vi "MoveROI.vi"(7 "Direction":enum16{"X+", "X-", "Y+", "Y-"}(ring), 8 "error in (no error)":errorcluster, 9 "Pitch":i32, 10 "ROI In":T1 {"Contours"."Type" items=["No Selection", "Point", "Line", "Rectangle", "Oval", "Polygon", "Freehand Region", "Annulus", "Unused2", "Unused3", "Broken Line", "Freehand Line", "Rotated Rectangle"]}) -> (0 "error out":errorcluster, 2 "ROI Out":T1 {"Contours"."Type" items=["No Selection", "Point", "Line", "Rectangle", "Oval", "Polygon", "Freehand Region", "Annulus", "Unused2", "Unused3", "Broken Line", "Freehand Line", "Rotated Rectangle"]})   [LabVIEW 2019]
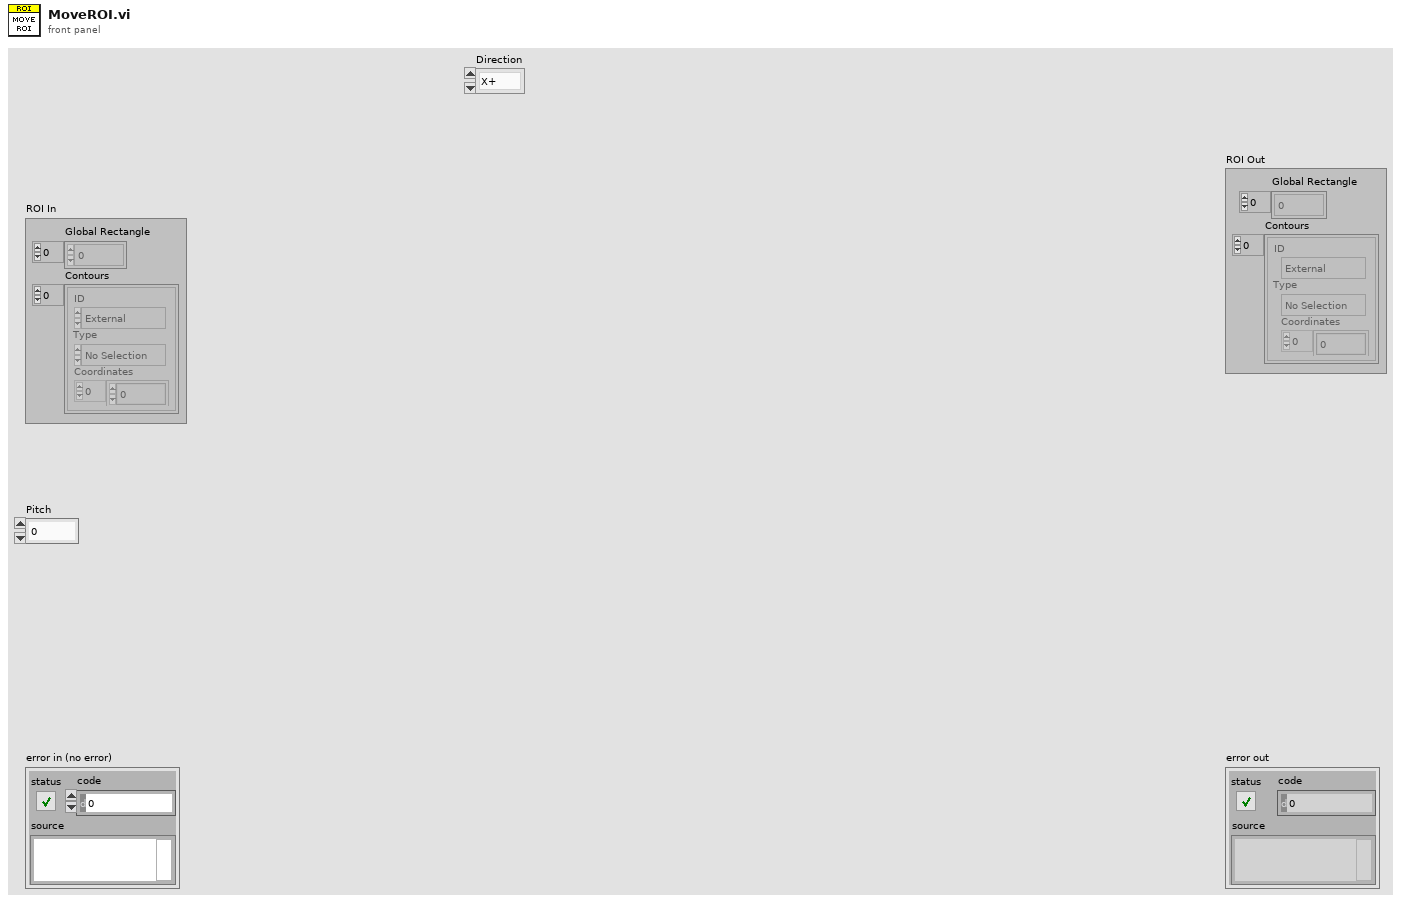
[diagram p1: front panel]
types:
  T1 = typedef "ROI Descriptor" = cluster{"Global Rectangle":i32[], "Contours":cluster{"ID":enum32{"External", "Internal"}, "Type":u32, "Coordinates":i32[]}[]}
  T2 = cluster{"ID":enum32{"External", "Internal"}, "Type":u32, "Coordinates":i32[]}[]
  T3 = cluster{"ID":enum32{"External", "Internal"}, "Type":u32, "Coordinates":i32[]}
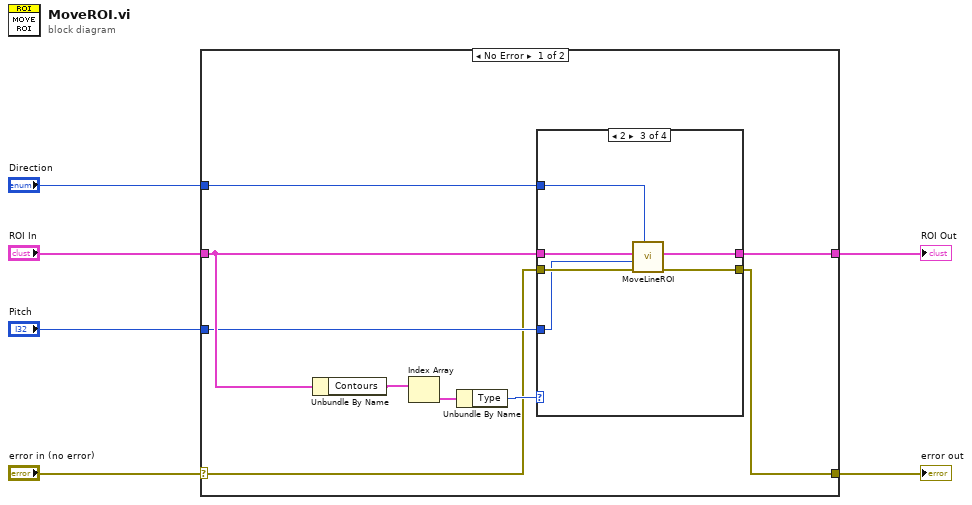
[diagram p0: block diagram]
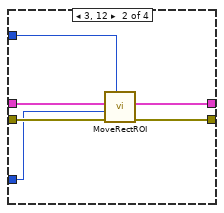
[diagram p3: hidden frame]
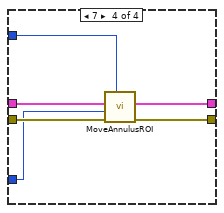
[diagram p4: hidden frame]
diagram:
  n1 = case shown="No Error" "error in (no error)" {
    selector: "error in (no error)" -> [w9 w37]
    tunnel: "ROI In" -> [w15 w36]
    tunnel: "Direction" -> [w11 _]
    tunnel: "Pitch" -> [w10 _]
    tunnel: [w8 w37] -> w2
    tunnel: [w7 w36] -> w1
    frame No Error {
      n2 = Unbundle By Name(w15) -> ("Contours"=w14:T2)
      n3 = Index Array(array=w14) -> (element=w13:T3)  [unwired: 1 in]
      n4 = Unbundle By Name(w13) -> ("Type"=w12:u32)
      n5 = case shown="2" w12 {
        tunnel: w11 -> [_ w18 w29 w33]
        tunnel: [w17 w23 w28 w35] -> w7
        tunnel: [w16 w22 w27 w34] -> w8
        tunnel: w15 -> [w17 w21 w25 w32]
        tunnel: w9 -> [w16 w20 w26 w31]
        tunnel: w10 -> [_ w19 w24 w30]
        frame Default {
        }
        frame 3, 12 {
          n6 = call "MoveRectROI.vi"("Action"=w18, "error in (no error)"=w20, "PItch"=w19, "ROI In"=w21) -> ("error out"=w22:errorcluster, "ROI Out"=w23:T1)  [unwired: 6 in]
        }
        frame 2 {
          n7 = call "MoveLineROI.vi"("Action"=w29, "error in (no error)"=w26, "PItch"=w24, "ROI In"=w25) -> ("error out"=w27:errorcluster, "ROI Out"=w28:T1)  [unwired: 6 in]
        }
        frame 7 {
          n8 = call "MoveAnnulusROI.vi"("Action"=w33, "error in (no error)"=w31, "PItch"=w30, "ROI In"=w32) -> ("error out"=w34:errorcluster, "ROI Out"=w35:T1)  [unwired: 6 in]
        }
      }
    }
    frame Error {
    }
  }
  "error out" <- w2
  "ROI Out" <- w1
